vi "Piano.vi"() -> ()   [LabVIEW 2023]
uses:
  <instrlib>/HandsOnPi2040/cti-drivers-lv-visa-main/CTI-Visa/Identity.ctl
  <instrlib>/HandsOnPi2040/Public/AOs.ctl
  <instrlib>/HandsOnPi2040/Public/PWMSettings.ctl
  <instrlib>/HandsOnPi2040/HandsOnPi2040.lvlib
  <instrlib>/HandsOnPi2040/cti-drivers-lv-visa-main/CTI-Visa/CTI-Visa.lvlib
panel:
  out "error out":errorcluster
  out "Identity":T1
  in  "Duty Cycle":dbl(slide)=0.09183673469387754 scale=0.0..1.0
  in  "D5#":bool
  in  "E5":bool
  in  "C5#":bool
  in  "D5":bool
  in  "A4#":bool
  in  "G4#":bool
  in  "F4#":bool
  in  "D4#":bool
  in  "C4#":bool
  in  "VISA resource":refnum<visa-resource-name>="ASRL5::INSTR"
  in  "stop":bool
  in  "C5":bool
  in  "B4":bool
  in  "A4":bool
  in  "G4":bool
  in  "F4":bool
  in  "E4":bool
  in  "D4":bool
  in  "C4":bool
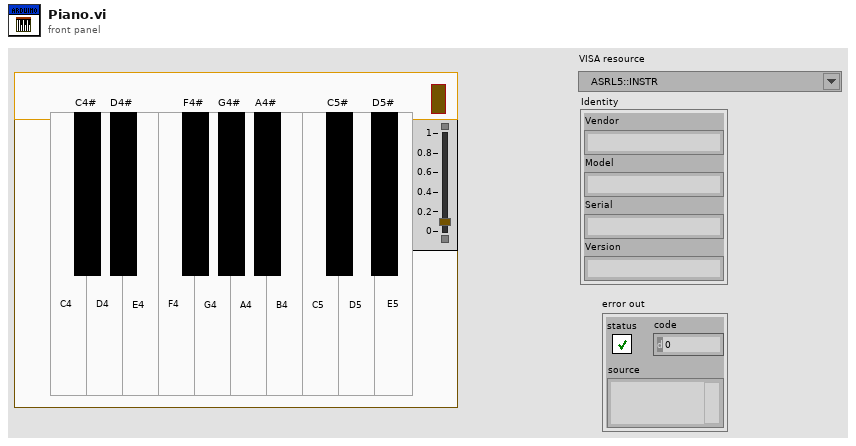
[diagram p1: front panel]
types:
  T1 = typedef "CTI-Visa.lvlib/Identity.ctl" = cluster{"Vendor":string, "Model":string, "Serial":string, "Version":string}
  T2 = typedef "HandsOnPi2040.lvlib/PWMSettings.ctl" = cluster{"Duty":sgl, "Frequency":sgl}
  T3 = typedef "HandsOnPi2040.lvlib/AOs.ctl" = enum16{"No AO - Error", "AO1 (GPIO28)"}
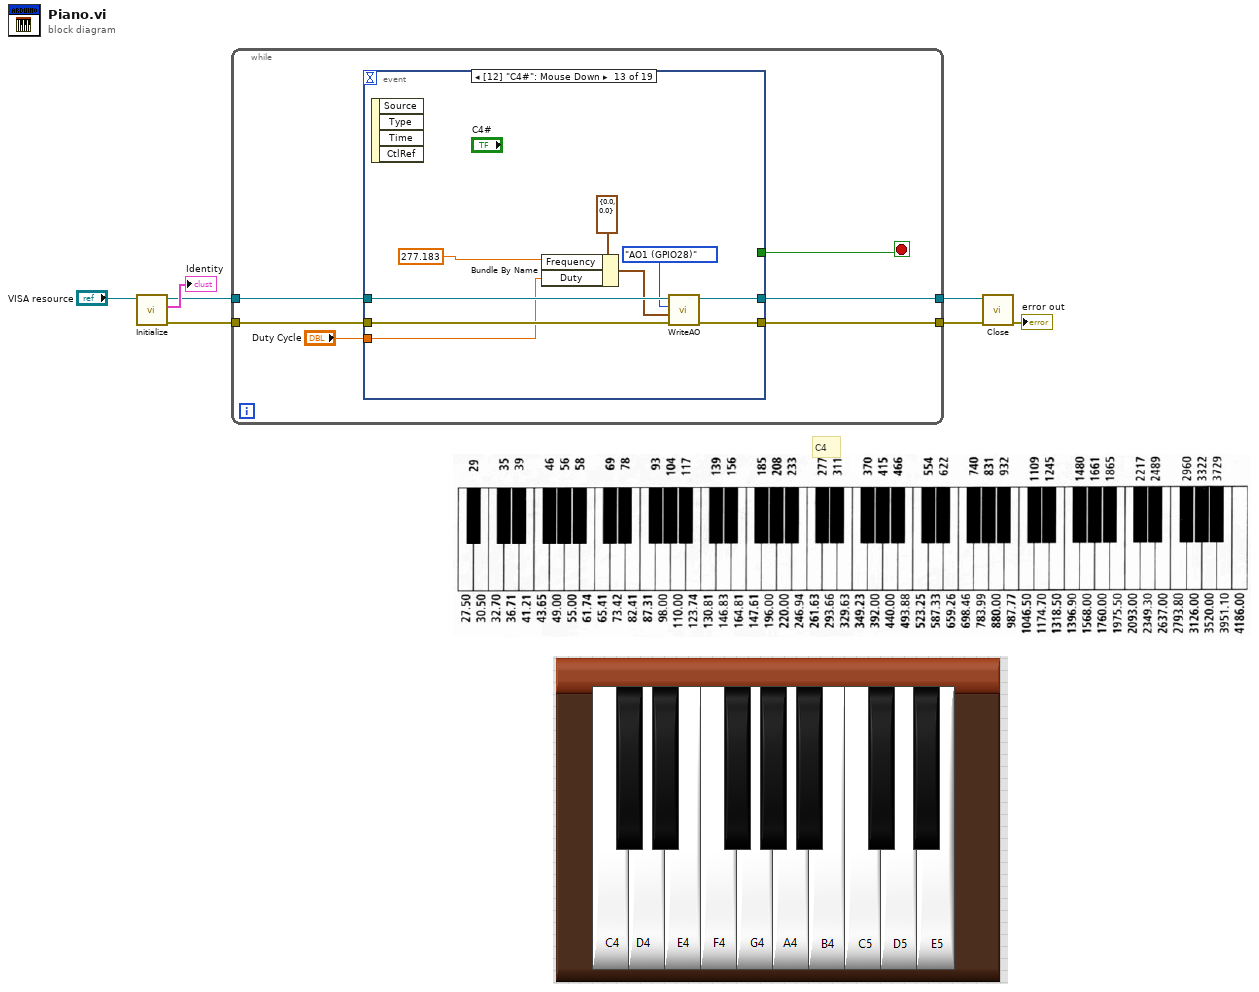
[diagram p0: block diagram]
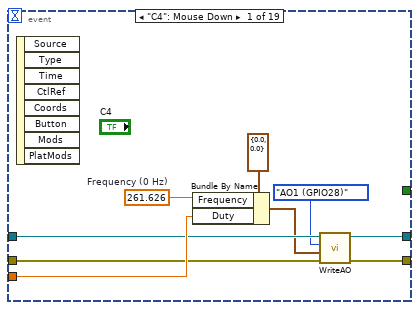
[diagram p2: hidden frame]
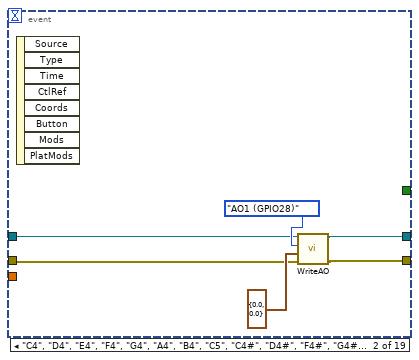
[diagram p3: hidden frame]
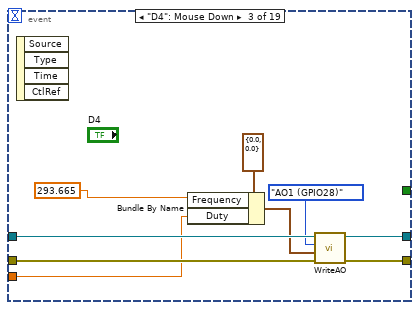
[diagram p4: hidden frame]
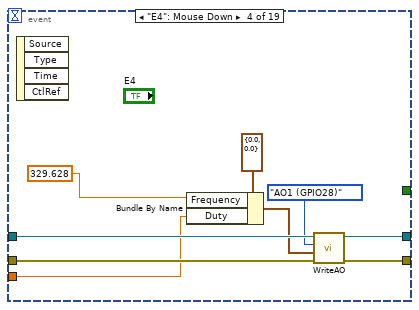
[diagram p5: hidden frame]
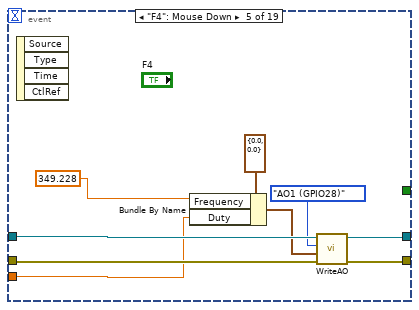
[diagram p6: hidden frame]
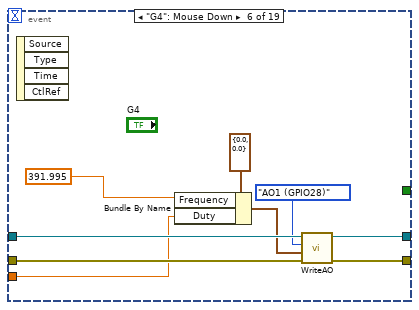
[diagram p7: hidden frame]
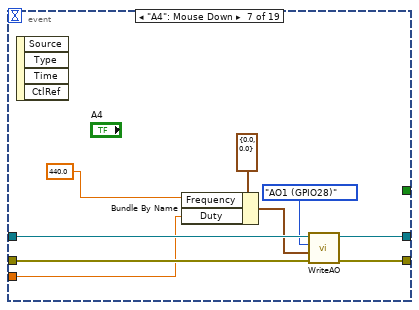
[diagram p8: hidden frame]
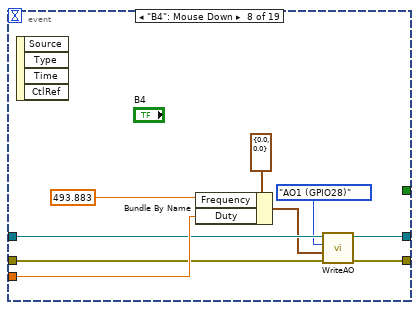
[diagram p9: hidden frame]
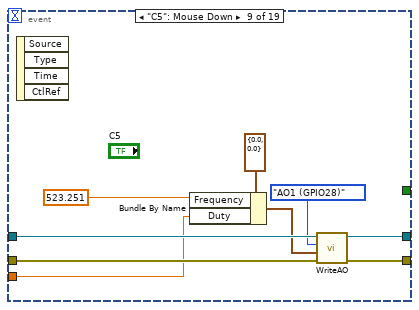
[diagram p10: hidden frame]
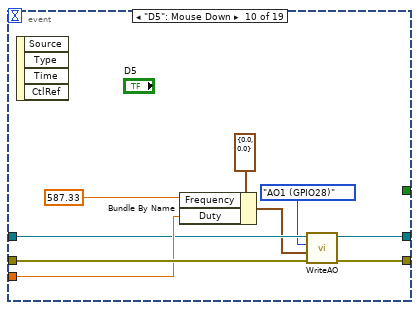
[diagram p11: hidden frame]
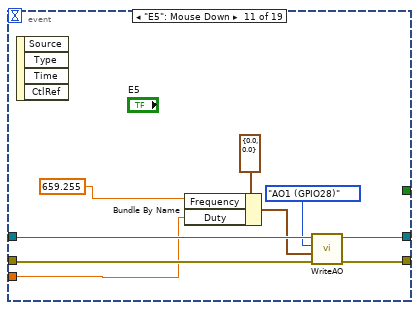
[diagram p12: hidden frame]
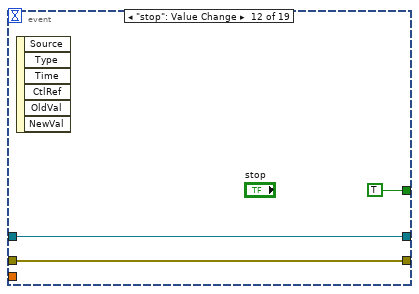
[diagram p13: hidden frame]
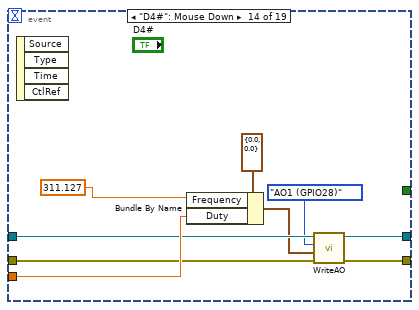
[diagram p14: hidden frame]
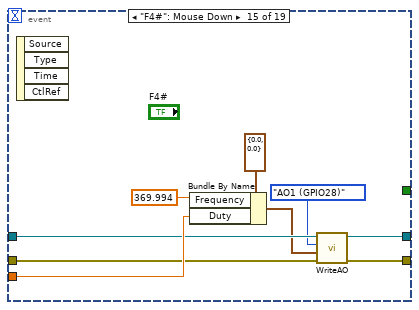
[diagram p15: hidden frame]
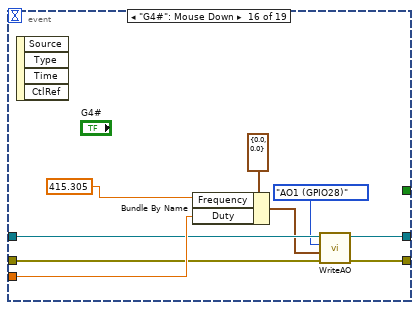
[diagram p16: hidden frame]
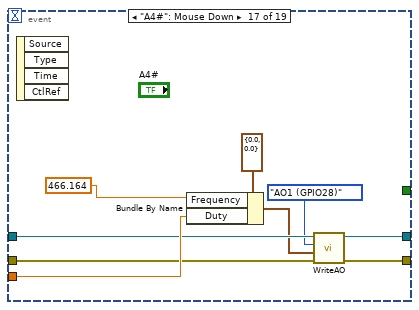
[diagram p17: hidden frame]
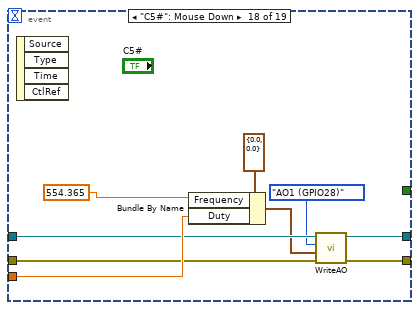
[diagram p18: hidden frame]
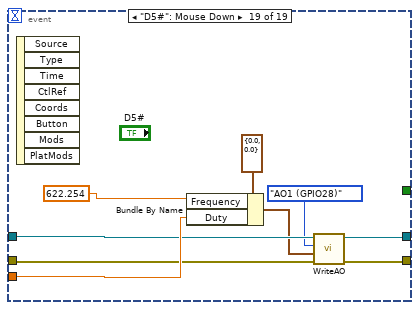
[diagram p19: hidden frame]
diagram:
  # "C4"
  n1 = call <instrlib>:"Initialize.vi"("VISA resource name"="VISA resource") -> ("error out"=w4:errorcluster, "Identity"=→"Identity":T1, "VISA resource name out"=w5:refnum<visa-resource-name>)  [unwired: 8 in]
  n2 = while {
    tunnel: w5 -> [w12]
    tunnel: w4 -> [w11]
    tunnel: [w8] -> w2
    tunnel: [w9] -> w1
    stop <- w10 stop-if-true
    n3 = event shown="[12] \"C4#\": Mouse Down" {
      selector: _ -> [_ _ _ _ _ _ _ _ _ _ _ _ _ _ _ _ _ _ _]
      dyn-events: _ -> [_ _ _ _ _ _ _ _ _ _ _ _ _ _ _ _ _ _ _]
      timeout: _ -> [_ _ _ _ _ _ _ _ _ _ _ _ _ _ _ _ _ _ _]
      tunnel: "Duty Cycle" -> [w20 _ w32 w42 w50 w60 w69 w82 w86 w97 w104 _ w117 w128 w137 w146 w155 w164 w173]
      tunnel: w12 -> [w18 w23 w34 w44 w52 w62 w71 w80 w88 w96 w106 w111 w118 w126 w135 w144 w153 w162 w171]
      tunnel: w11 -> [w19 w24 w33 w43 w51 w61 w70 w81 w89 w98 w105 w110 w119 w127 w136 w145 w154 w163 w172]
      tunnel: [w21 w25 w36 w45 w54 w64 w72 w79 w90 w99 w108 w110 w120 w130 w138 w147 w157 w165 w174] -> w8
      tunnel: [w22 w26 w37 w46 w55 w63 w73 w78 w91 w100 w107 w111 w121 w129 w139 w148 w156 w166 w175] -> w9
      tunnel: [_ _ _ _ _ _ _ _ _ _ _ TRUE _ _ _ _ _ _ _] -> w10
      event "C4": Mouse Down {
        w17 = 261.626  # Frequency (0 Hz)
        n4 = event-data() -> ()  [unwired: 1 in, 8 out]
        n5 = Bundle By Name(cluster=T2 {"Duty"=0.0, "Frequency"=0.0} ("PWM Settings"), "Frequency"=w17, "Duty"=w20) -> (w14:T2)
        n6 = call <instrlib>:"WriteAO.vi"("error in (no error)"=w19, "PWM Settings"=w14, "Analog Output"=AOs."AO1 (GPIO28)", "VISA resource name"=w18) -> ("error out"=w21:errorcluster, "VISA resource name out"=w22:refnum<visa-resource-name>)  [unwired: 6 in]
      }
      event "C4", "D4", "E4", "F4", "G4", "A4", "B4", "C5", "C4#", "D4#", "F4#", "G4#", "A4#", "C5#", "D5", "D5#", "E5": Mouse Up {
        n7 = event-data() -> ()  [unwired: 1 in, 8 out]
        n8 = call <instrlib>:"WriteAO.vi"("error in (no error)"=w24, "PWM Settings"=T2 {"Duty"=0.0, "Frequency"=0.0}, "Analog Output"=AOs."AO1 (GPIO28)", "VISA resource name"=w23) -> ("error out"=w25:errorcluster, "VISA resource name out"=w26:refnum<visa-resource-name>)  [unwired: 6 in]
      }
      event "D4": Mouse Down {
        n9 = event-data() -> ()  [unwired: 1 in, 4 out]
        n10 = Bundle By Name(cluster=T2 {"Duty"=0.0, "Frequency"=0.0} ("PWM Settings"), "Frequency"=293.665 ("Frequency (0 Hz)"), "Duty"=w32) -> (w29:T2)
        n11 = call <instrlib>:"WriteAO.vi"("error in (no error)"=w33, "PWM Settings"=w29, "Analog Output"=AOs."AO1 (GPIO28)", "VISA resource name"=w34) -> ("error out"=w36:errorcluster, "VISA resource name out"=w37:refnum<visa-resource-name>)  [unwired: 6 in]
      }
      event "E4": Mouse Down {
        n12 = event-data() -> ()  [unwired: 1 in, 4 out]
        n13 = Bundle By Name(cluster=T2 {"Duty"=0.0, "Frequency"=0.0} ("PWM Settings"), "Frequency"=329.628 ("Frequency (0 Hz)"), "Duty"=w42) -> (w38:T2)
        n14 = call <instrlib>:"WriteAO.vi"("error in (no error)"=w43, "PWM Settings"=w38, "Analog Output"=AOs."AO1 (GPIO28)", "VISA resource name"=w44) -> ("error out"=w45:errorcluster, "VISA resource name out"=w46:refnum<visa-resource-name>)  [unwired: 6 in]
      }
      event "F4": Mouse Down {
        n15 = event-data() -> ()  [unwired: 1 in, 4 out]
        n16 = Bundle By Name(cluster=T2 {"Duty"=0.0, "Frequency"=0.0} ("PWM Settings"), "Frequency"=349.228, "Duty"=w50) -> (w47:T2)
        n17 = call <instrlib>:"WriteAO.vi"("error in (no error)"=w51, "PWM Settings"=w47, "Analog Output"=AOs."AO1 (GPIO28)", "VISA resource name"=w52) -> ("error out"=w54:errorcluster, "VISA resource name out"=w55:refnum<visa-resource-name>)  [unwired: 6 in]
      }
      event "G4": Mouse Down {
        n18 = event-data() -> ()  [unwired: 1 in, 4 out]
        n19 = Bundle By Name(cluster=T2 {"Duty"=0.0, "Frequency"=0.0} ("PWM Settings"), "Frequency"=391.995, "Duty"=w60) -> (w56:T2)
        n20 = call <instrlib>:"WriteAO.vi"("error in (no error)"=w61, "PWM Settings"=w56, "Analog Output"=AOs."AO1 (GPIO28)", "VISA resource name"=w62) -> ("error out"=w64:errorcluster, "VISA resource name out"=w63:refnum<visa-resource-name>)  [unwired: 6 in]
      }
      event "A4": Mouse Down {
        n21 = event-data() -> ()  [unwired: 1 in, 4 out]
        n22 = Bundle By Name(cluster=T2 {"Duty"=0.0, "Frequency"=0.0} ("PWM Settings"), "Frequency"=440.0, "Duty"=w69) -> (w65:T2)
        n23 = call <instrlib>:"WriteAO.vi"("error in (no error)"=w70, "PWM Settings"=w65, "Analog Output"=AOs."AO1 (GPIO28)", "VISA resource name"=w71) -> ("error out"=w72:errorcluster, "VISA resource name out"=w73:refnum<visa-resource-name>)  [unwired: 6 in]
      }
      event "B4": Mouse Down {
        n24 = event-data() -> ()  [unwired: 1 in, 4 out]
        n25 = Bundle By Name(cluster=T2 {"Duty"=0.0, "Frequency"=0.0} ("PWM Settings"), "Frequency"=493.883, "Duty"=w82) -> (w74:T2)
        n26 = call <instrlib>:"WriteAO.vi"("error in (no error)"=w81, "PWM Settings"=w74, "Analog Output"=AOs."AO1 (GPIO28)", "VISA resource name"=w80) -> ("error out"=w79:errorcluster, "VISA resource name out"=w78:refnum<visa-resource-name>)  [unwired: 6 in]
      }
      event "C5": Mouse Down {
        n27 = event-data() -> ()  [unwired: 1 in, 4 out]
        n28 = Bundle By Name(cluster=T2 {"Duty"=0.0, "Frequency"=0.0} ("PWM Settings"), "Frequency"=523.251, "Duty"=w86) -> (w83:T2)
        n29 = call <instrlib>:"WriteAO.vi"("error in (no error)"=w89, "PWM Settings"=w83, "Analog Output"=AOs."AO1 (GPIO28)", "VISA resource name"=w88) -> ("error out"=w90:errorcluster, "VISA resource name out"=w91:refnum<visa-resource-name>)  [unwired: 6 in]
      }
      event "D5": Mouse Down {
        n30 = event-data() -> ()  [unwired: 1 in, 4 out]
        n31 = Bundle By Name(cluster=T2 {"Duty"=0.0, "Frequency"=0.0} ("PWM Settings"), "Frequency"=587.33, "Duty"=w97) -> (w92:T2)
        n32 = call <instrlib>:"WriteAO.vi"("error in (no error)"=w98, "PWM Settings"=w92, "Analog Output"=AOs."AO1 (GPIO28)", "VISA resource name"=w96) -> ("error out"=w99:errorcluster, "VISA resource name out"=w100:refnum<visa-resource-name>)  [unwired: 6 in]
      }
      event "E5": Mouse Down {
        n33 = event-data() -> ()  [unwired: 1 in, 4 out]
        n34 = Bundle By Name(cluster=T2 {"Duty"=0.0, "Frequency"=0.0} ("PWM Settings"), "Frequency"=659.255, "Duty"=w104) -> (w101:T2)
        n35 = call <instrlib>:"WriteAO.vi"("error in (no error)"=w105, "PWM Settings"=w101, "Analog Output"=AOs."AO1 (GPIO28)", "VISA resource name"=w106) -> ("error out"=w108:errorcluster, "VISA resource name out"=w107:refnum<visa-resource-name>)  [unwired: 6 in]
      }
      event "stop": Value Change {
        n36 = event-data() -> ()  [unwired: 1 in, 6 out]
      }
      event "C4#": Mouse Down {
        n37 = event-data() -> ()  [unwired: 1 in, 4 out]
        n38 = Bundle By Name(cluster=T2 {"Duty"=0.0, "Frequency"=0.0} ("PWM Settings"), "Frequency"=277.183, "Duty"=w117) -> (w113:T2)
        n39 = call <instrlib>:"WriteAO.vi"("error in (no error)"=w119, "PWM Settings"=w113, "Analog Output"=AOs."AO1 (GPIO28)", "VISA resource name"=w118) -> ("error out"=w120:errorcluster, "VISA resource name out"=w121:refnum<visa-resource-name>)  [unwired: 6 in]
      }
      event "D4#": Mouse Down {
        n40 = event-data() -> ()  [unwired: 1 in, 4 out]
        n41 = Bundle By Name(cluster=T2 {"Duty"=0.0, "Frequency"=0.0} ("PWM Settings"), "Frequency"=311.127, "Duty"=w128) -> (w122:T2)
        n42 = call <instrlib>:"WriteAO.vi"("error in (no error)"=w127, "PWM Settings"=w122, "Analog Output"=AOs."AO1 (GPIO28)", "VISA resource name"=w126) -> ("error out"=w130:errorcluster, "VISA resource name out"=w129:refnum<visa-resource-name>)  [unwired: 6 in]
      }
      event "F4#": Mouse Down {
        n43 = event-data() -> ()  [unwired: 1 in, 4 out]
        n44 = Bundle By Name(cluster=T2 {"Duty"=0.0, "Frequency"=0.0} ("PWM Settings"), "Frequency"=369.994, "Duty"=w137) -> (w131:T2)
        n45 = call <instrlib>:"WriteAO.vi"("error in (no error)"=w136, "PWM Settings"=w131, "Analog Output"=AOs."AO1 (GPIO28)", "VISA resource name"=w135) -> ("error out"=w138:errorcluster, "VISA resource name out"=w139:refnum<visa-resource-name>)  [unwired: 6 in]
      }
      event "G4#": Mouse Down {
        n46 = event-data() -> ()  [unwired: 1 in, 4 out]
        n47 = Bundle By Name(cluster=T2 {"Duty"=0.0, "Frequency"=0.0} ("PWM Settings"), "Frequency"=415.305, "Duty"=w146) -> (w140:T2)
        n48 = call <instrlib>:"WriteAO.vi"("error in (no error)"=w145, "PWM Settings"=w140, "Analog Output"=AOs."AO1 (GPIO28)", "VISA resource name"=w144) -> ("error out"=w147:errorcluster, "VISA resource name out"=w148:refnum<visa-resource-name>)  [unwired: 6 in]
      }
      event "A4#": Mouse Down {
        n49 = event-data() -> ()  [unwired: 1 in, 4 out]
        n50 = Bundle By Name(cluster=T2 {"Duty"=0.0, "Frequency"=0.0} ("PWM Settings"), "Frequency"=466.164, "Duty"=w155) -> (w149:T2)
        n51 = call <instrlib>:"WriteAO.vi"("error in (no error)"=w154, "PWM Settings"=w149, "Analog Output"=AOs."AO1 (GPIO28)", "VISA resource name"=w153) -> ("error out"=w157:errorcluster, "VISA resource name out"=w156:refnum<visa-resource-name>)  [unwired: 6 in]
      }
      event "C5#": Mouse Down {
        n52 = event-data() -> ()  [unwired: 1 in, 4 out]
        n53 = Bundle By Name(cluster=T2 {"Duty"=0.0, "Frequency"=0.0} ("PWM Settings"), "Frequency"=554.365, "Duty"=w164) -> (w158:T2)
        n54 = call <instrlib>:"WriteAO.vi"("error in (no error)"=w163, "PWM Settings"=w158, "Analog Output"=AOs."AO1 (GPIO28)", "VISA resource name"=w162) -> ("error out"=w165:errorcluster, "VISA resource name out"=w166:refnum<visa-resource-name>)  [unwired: 6 in]
      }
      event "D5#": Mouse Down {
        n55 = event-data() -> ()  [unwired: 1 in, 8 out]
        n56 = Bundle By Name(cluster=T2 {"Duty"=0.0, "Frequency"=0.0} ("PWM Settings"), "Frequency"=622.254, "Duty"=w173) -> (w167:T2)
        n57 = call <instrlib>:"WriteAO.vi"("error in (no error)"=w172, "PWM Settings"=w167, "Analog Output"=AOs."AO1 (GPIO28)", "VISA resource name"=w171) -> ("error out"=w174:errorcluster, "VISA resource name out"=w175:refnum<visa-resource-name>)  [unwired: 6 in]
      }
    }
  }
  n58 = call <instrlib>:"Close.vi"("error in (no error)"=w2, "VISA resource name"=w1) -> ("error out"=→"error out":errorcluster)  [unwired: 9 in]
